vi "pp3_stateToDOInt.vi"(11 "State In":T1={"Curr  tr"=0, "Curr (ms)"=0, "Cum (ms)"=0, "Run loop diff"=0, "Tone countdown (ms)"=0, "Countdown (ms)"=0, "Curr State"=enum."0 NULL", "Prev State"=enum."0 NULL", "Rw"=FALSE, "Sw"=FALSE, "Tone\nGate"=FALSE, "Punish"=FALSE, "Current DAQ DO Int"=0, "Current Loaded Trial"={"Trial Type Number"=1, "Trial Type"=enum."GO", "Trial Weight"=100, "Shock (mA)"=0.3, "Duration (ms)"=0.25, "Sound Type"=enum."04 FM Sweep", "Stim P1"=4000.0, "Stim P2"=0.0, "Stim P3"=0.0, "Stim P4"=2000.0, "DAQ Amplitude (V)"=0.25}, "Total trials memo"=0, "State start cum memo (ms)"=0, "Last dur jump time memo (ms)"=0, "Last dur shock time memo (ms)"=0, "Tone repeat memo (ms)"=0, "Webcam on"=FALSE, "Webcam recording"=FALSE, "State update flag"=FALSE, "Last loaded shock voltage"=0.0, "Vid upd"=enum."0", "First time tone"=FALSE} {"Current DAQ DO Int" format="%016b"; "Current Loaded Trial"."DAQ Amplitude (V)" min=0.0 max=5.0 format="%_4g"; "Current Loaded Trial"."Shock (mA)" min=-1.0 max=5.0; "Current Loaded Trial"."Trial Weight" step=1; "Current Loaded Trial"."Duration (ms)" min=0.0 max=1.0; "Current Loaded Trial"."Trial Type Number" min=1 max=256 step=1}) -> (3 "DAQ Output Int":u16 format="%016b")   [LabVIEW 2013]
uses:
  CTL_pp3c_LoopState.ctl
  pp3_CTL_BehavioralState.ctl
  pp3_CTL_Trial.ctl
  pp3_CTL_TrialType.ctl
  labolabo2/waveforms/WFTypes.ctl
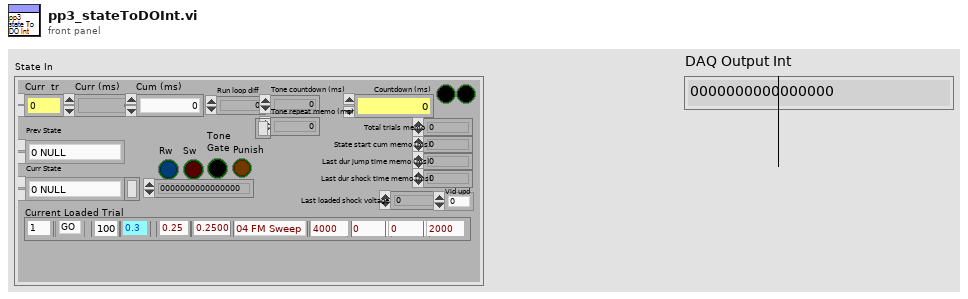
[diagram p1: front panel]
types:
  T1 = typedef "CTL_pp3c_LoopState.ctl" = cluster{"Curr  tr":u16, "Curr (ms)":u32, "Cum (ms)":u64, "Run loop diff":i64, "Tone countdown (ms)":i64, "Countdown (ms)":i64, "Curr State":T2, "Prev State":T2, "Rw":bool, "Sw":bool, "Tone\nGate":bool, "Punish":bool, "Current DAQ DO Int":u16, "Current Loaded Trial":T3, "Total trials memo":i64, "State start cum memo (ms)":i64, "Last dur jump time memo (ms)":i64, "Last dur shock time memo (ms)":i64, "Tone repeat memo (ms)":i64, "Webcam on":bool, "Webcam recording":bool, "State update flag":bool, "Last loaded shock voltage":dbl, "Vid upd":enum16{"0", "1", "2", "3", "4", "5", "6", "7", "8", "9"}, "First time tone":bool}
  T2 = typedef "pp3_CTL_BehavioralState.ctl" = enum8{"0 NULL", "1 Habituation", "2 (Load Trial)", "3 Stay Period", "4 Load Audio/Click Delay", "5 GO Trial", "6 GO Jumped", "7 GO Timeout", "8 NOGO Trial", "9 NOGO Jumped", "10 NOGO Timeout", "11 TEST Trial", "12 TEST Jumped", "13 TEST Timeout", "14 Intertrial Interval", "15 Done"}
  T3 = typedef "pp3_CTL_Trial.ctl" = cluster{"Trial Type Number":i16, "Trial Type":T4, "Trial Weight":u32, "Shock (mA)":dbl, "Duration (ms)":dbl, "Sound Type":T5, "Stim P1":dbl, "Stim P2":dbl, "Stim P3":dbl, "Stim P4":dbl, "DAQ Amplitude (V)":dbl}
  T4 = typedef "pp3_CTL_TrialType.ctl" = enum16{"OFF", "GO", "NOGO", "TEST"}
  T5 = typedef "WFTypes.ctl" = enum16{"00 NULL", "01 DC", "02 Noise", "03 Pure Tone", "04 FM Sweep"}
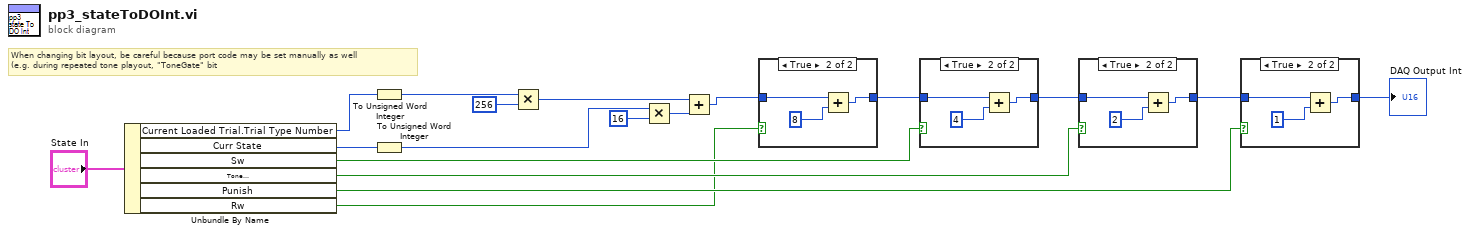
[diagram p0: block diagram]
diagram:
  # "When changing bit layout, be careful because port code may be set manually as well\n(e.g. during repeated tone playout, \"ToneGate\" bit"
  n1 = Unbundle By Name("State In") -> ("Current Loaded Trial.Trial Type Number"=w16:i16, "Curr State"=w4:T2, "Sw"=w5:bool, "Tone\nGate"=w7:bool, "Punish"=w8:bool, "Rw"=w1:bool)
  n2 = To Unsigned Word Integer(number=w16) -> (unsigned 16bit integer=w15:u16)
  n3 = To Unsigned Word Integer(number=w4) -> (unsigned 16bit integer=w11:u16)
  n4 = Multiply(x=w15, y=u16 256) -> (x*y=w10:u16)
  n5 = Multiply(x=w11, y=u16 16) -> (x*y=w9:u16)
  n6 = Add(x=w10, y=w9) -> (x+y=w2:u16)
  n7 = case shown="True" w1 {
    tunnel: [w19 w21] -> w3
    tunnel: w2 -> [w19 w20]
    frame False {
    }
    frame True {
      n8 = Add(x=w20, y=u16 8 ("Current DAQ Digital Out")) -> (x+y=w21:u16)
    }
  }
  n9 = case shown="True" w5 {
    tunnel: [w23 w25] -> w14
    tunnel: w3 -> [w23 w24]
    frame False {
    }
    frame True {
      n10 = Add(x=w24, y=u16 4 ("Current DAQ Digital Out")) -> (x+y=w25:u16)
    }
  }
  n11 = case shown="True" w7 {
    tunnel: w14 -> [w27 w29]
    tunnel: [w27 w28] -> w13
    frame False {
    }
    frame True {
      n12 = Add(x=w29, y=u16 2 ("Current DAQ Digital Out")) -> (x+y=w28:u16)
    }
  }
  n13 = case shown="True" w8 {
    tunnel: w13 -> [w31 w33]
    tunnel: [w31 w32] -> w6
    frame False {
    }
    frame True {
      n14 = Add(x=w33, y=u16 1 ("Current DAQ Digital Out")) -> (x+y=w32:u16)
    }
  }
  "DAQ Output Int" <- w6
